vi "CompareTrackerBiasZ.vi"() -> ()   [LabVIEW 2011]
uses:
  qtrk/QTrkLVBinding/XYZf.ctl
  qtrk/lv/CPUTrkAPI.llb/TrackerDLL.vi
panel:
  out "LV LUT size":i32[](array[numeric])
  out "iz":T1(graph)
  out "iz-z":T2(graph)
  out "Error curves":dbl[][](graph)
  out "LV BestIndex":i32
  out "QTrk bestIndex":i32
  out "Profiles":sgl[][](graph)
  in  "FFT Z compare?":bool
  out "X":T2(graph)
  out "LV LUT":dbl[][](graph)
  in  "file (use dialog)":path=path "D:/jcnossen1/datasets/refbeadmagtestlutpos/experim/rotation+forceramp/exp_qi.radialzlut"
  in  "LUT":sgl[][][](array[numeric])
  out "Z":T2(graph)
  out "Z":dbl[][](graph)
  out "Image":sgl[][](graph)
  out "X":dbl[][](graph)
  out "iteration":i32
  out "Intensity Graph":sgl[][](graph)
  in  "tracker DLL path":path=path "D:/jcnossen1/cudaqi-tracker/qtrk/lv/qtrk-labview.dll"
  in  "# images":i32=1000
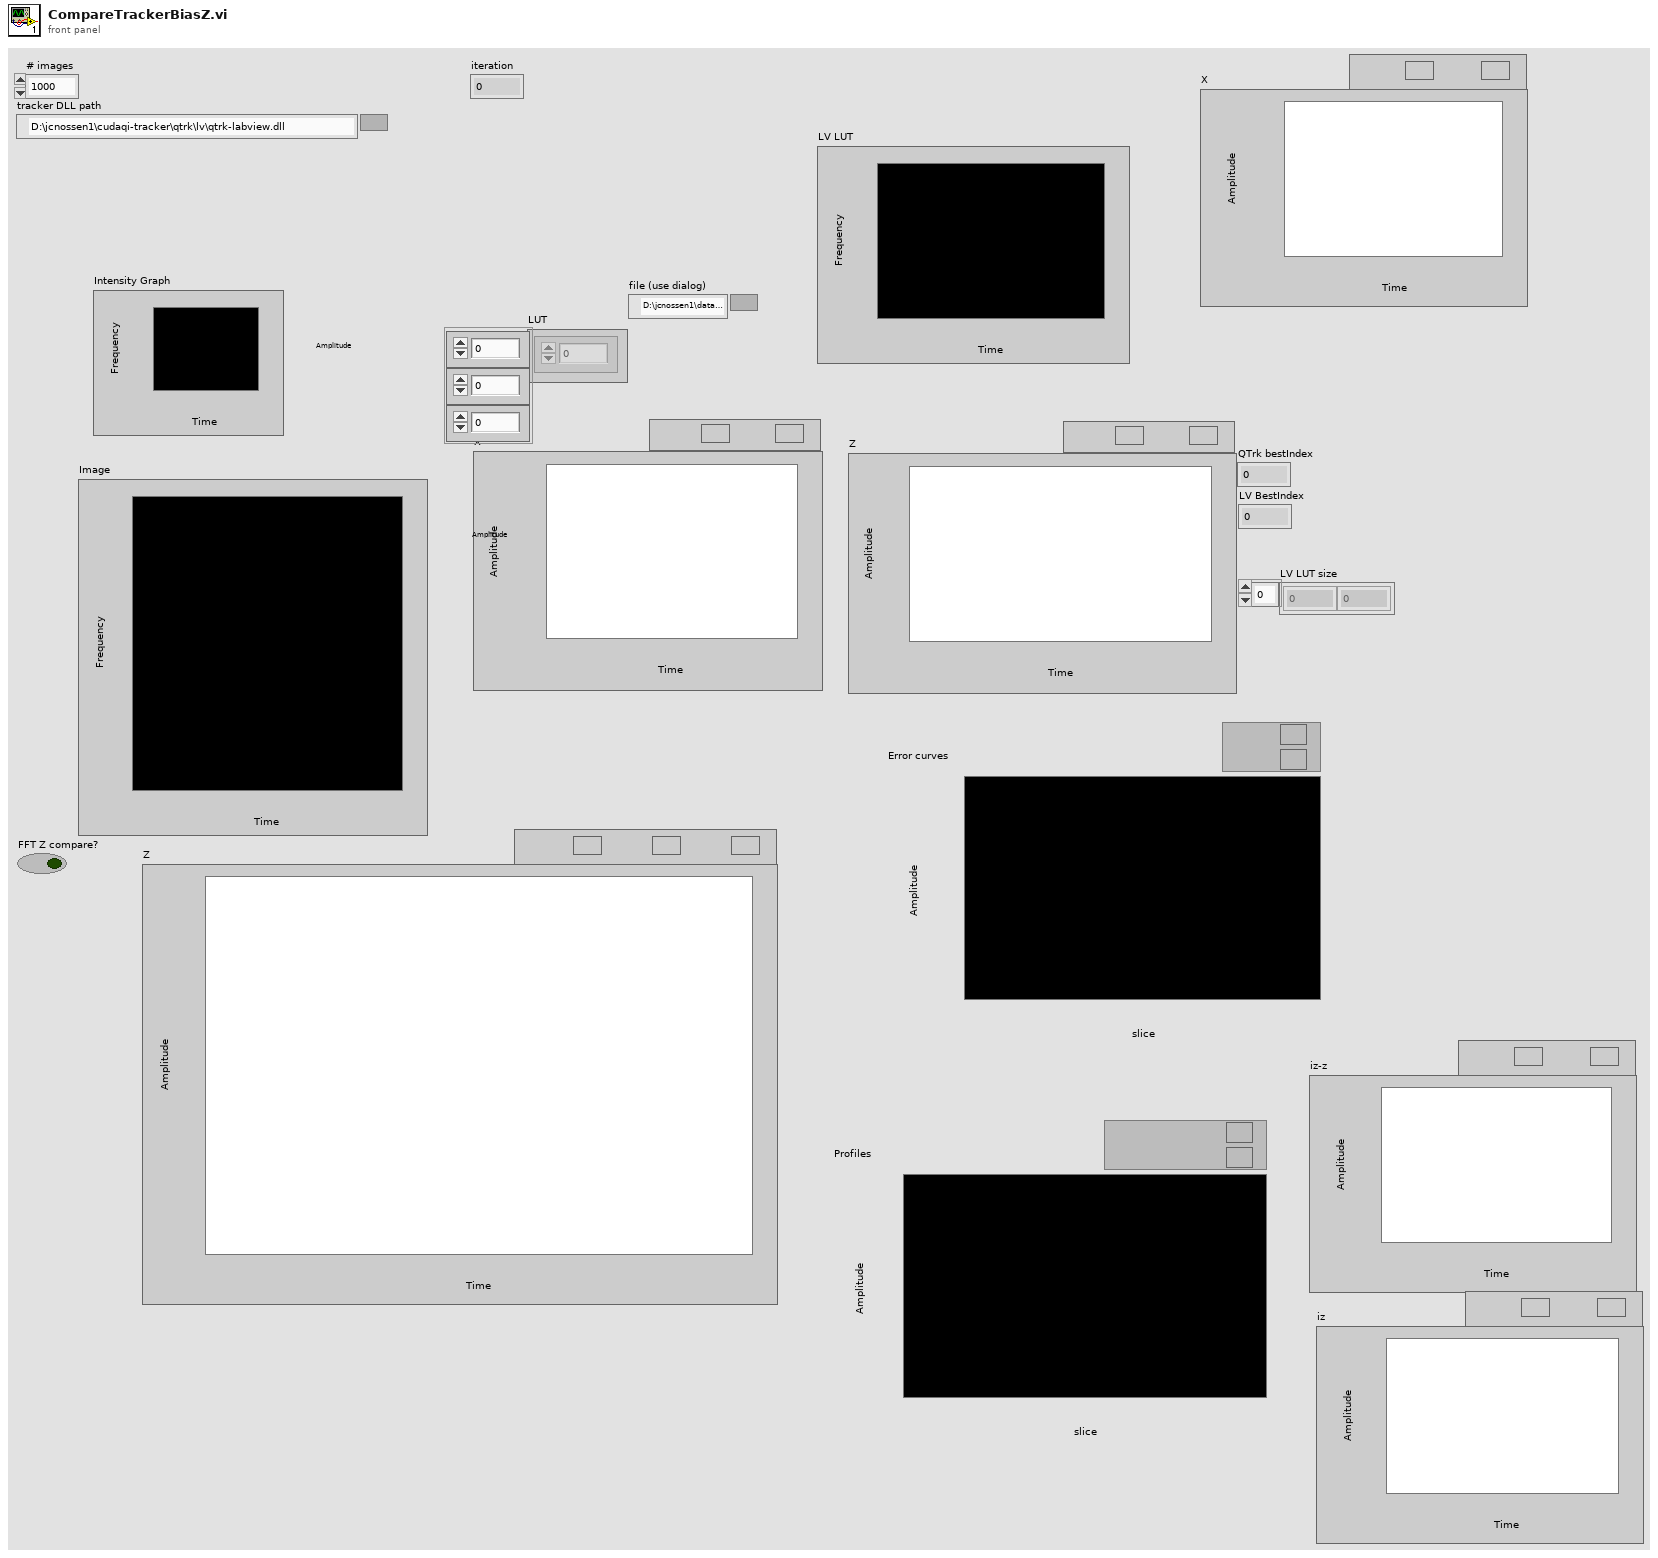
[diagram p1: front panel]
types:
  T1 = cluster{"[0]":i32, "[1]":i32, "[2]":i32, "[3]":i32, "[4]":i32, "[5]":i32, "[6]":i32, "[7]":i32, "[8]":i32}
  T2 = cluster{"[0]":dbl, "[1]":dbl, "[2]":dbl, "[3]":dbl, "[4]":dbl, "[5]":dbl, "[6]":dbl, "[7]":dbl, "[8]":dbl}
  T3 = enum16{"big-endian, network order", "native, host order", "little-endian"}
  T4 = typedef "TrackerInstance.ctl" = cluster{"Tracker Pointer":u64, "Image size":cluster{"width":u32, "height":u32}}
  T5 = cluster{"Rmax (pix)":i32, "RminZ (pix)":i32, "angular pixel\n coverage factor":dbl, "radial pixel\n coverage factor":dbl}
  T6 = typedef "XYZf.ctl" = cluster{"X":sgl, "Y":sgl, "Z":sgl}
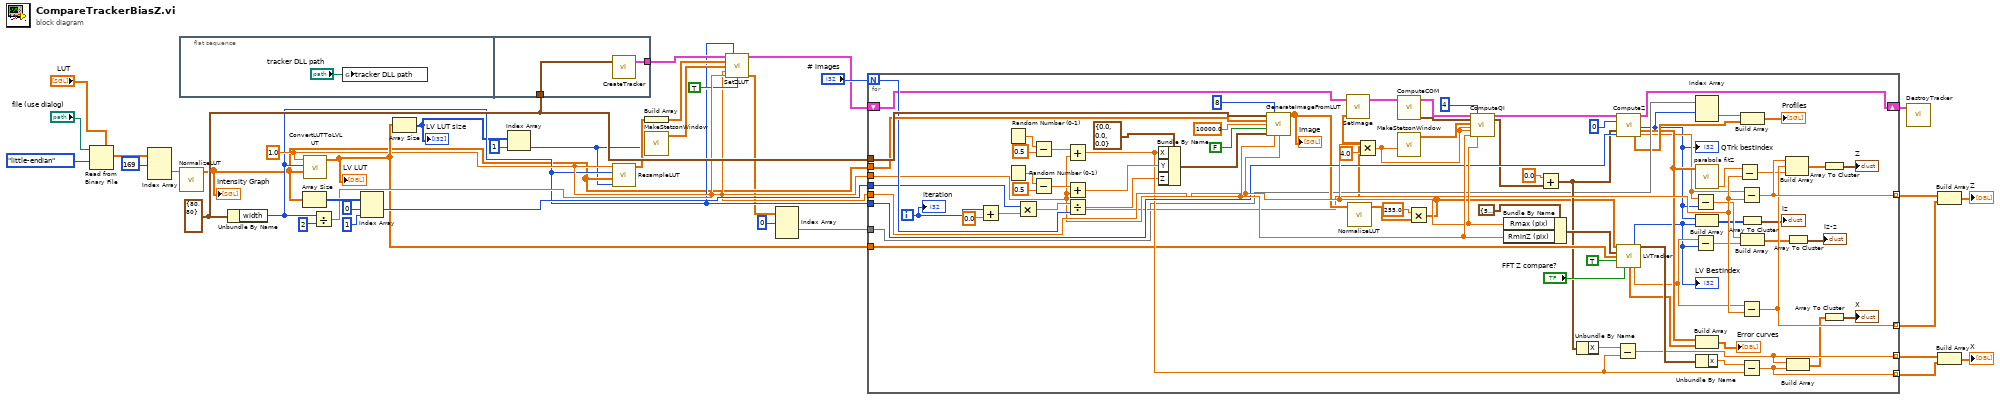
[diagram p0: block diagram]
diagram:
  w8 = sgl 1.0 ("minRadius")
  w16 = cluster{"width":u32, "height":u32} {"width"=80, "height"=80} ("Image size")
  n1 = Read from Binary File(5:"LUT", 9:T3."little-endian" ("byte order (0:big-endian, network order)"), 11:"file (use dialog)") -> (2:w19:sgl[][][])  [unwired: 3 in, 3 out]
  n2 = Index Array(array=w19, index (dim 0)=169 ("index (page)")) -> (element=w14:sgl[][])  [unwired: 2 in]
  n3 = flat-sequence {
    tunnel: [w40] -> w31
    tunnel: w16 -> [w39]
    frame #0 {
      n4 = global write "TrackerDLL.vi" "tracker DLL path"("tracker DLL path") -> ()
    }
    frame #1 {
      n5 = call "CreateTracker.vi"("Image size"=w39) -> ("tracker"=w40:T4)  [unwired: 2 in]
    }
  }
  n6 = call "NormalizeLUT.vi"("LUT"=w14) -> ("Array"=w4:sgl[][])  [unwired: 10 in]
  "Intensity Graph" <- w4
  n7 = Unbundle By Name(w16) -> ("width"=w7:u32)
  n8 = Array Size(array=w4) -> (size(s)=w35:i32[])
  n9 = call "ConvertLUTToLVLUT.vi"("LUT"=w4, "width"=w7, "minRadius"=w8) -> ("LV tracker rad prof"=w9:dbl[][])  [unwired: 8 in]
  "LV LUT" <- w9
  n10 = Divide(x=w7, y=u32 2) -> (x/y=w15:dbl)
  n11 = Index Array(array=w35, index #1=0 ("index"), index #2=1 ("index")) -> (element #1=w33:i32)  [unwired: 1 out]
  n12 = Array Size(array=w9) -> (size(s)=w6:i32[])
  "LV LUT size" <- w6
  n13 = Index Array(array=w6, index=1) -> (element=w2:i32)
  n14 = call "ResampleLUT.vi"("radialsteps"=w2, "LUT"=w4, "width"=w7, "minRadius"=w8) -> ("LUT"=w3:dbl[][])  [unwired: 7 in]
  n15 = Build Array(w3) -> (w13:dbl[][][])
  n16 = call "MakeStetsonWindow.vi"("radialsteps"=w2) -> ("Window"=w17:dbl[])  [unwired: 10 in]
  n17 = call "SetZLUT.vi"("tracker instance"=w31, "angularSteps"=w7, "zluts"=w13, "Radial weights"=w17, "minradius"=w8, "maxradius"=w15, "Normalize"=TRUE) -> ("tracker"=w30:T4, "normalized zlut"=w1:sgl[][][])  [unwired: 7 in]
  n18 = Index Array(array=w1, index (dim 0)=0 ("index (page)")) -> (element=w11:sgl[][])  [unwired: 2 in]
  n19 = for {
    N: "# images" -> [w113]
    tunnel: w16 -> [w118]
    tunnel: w4 -> [w117]
    tunnel: w15 -> [w86]
    tunnel: w33 -> [w94]
    shift-right: [w83] -> w32
    shift-left: w30 -> [w109]
    tunnel: [w70] -> w26 mode=indexing
    tunnel: [w60] -> w28 mode=indexing
    tunnel: w8 -> [w93]
    tunnel: w7 -> [w81]
    tunnel: [w79] -> w25 mode=indexing
    tunnel: [w78] -> w24 mode=indexing
    tunnel: w9 -> [w72]
    tunnel: w11 -> [w58]
    i -> [w112]
    n20 = Add(x=w112, y=0.0 ("X Range")) -> (x+y=w110:dbl)
    n21 = Random Number (0-1)() -> (number: 0 to 1=w92:dbl)
    n22 = Random Number (0-1)() -> (number: 0 to 1=w89:dbl)
    n23 = Multiply(x=w94, y=w110) -> (x*y=w114:dbl)
    n24 = Subtract(x=w92, y=0.5) -> (x-y=w90:dbl)
    n25 = Subtract(x=w89, y=0.5) -> (x-y=w87:dbl)
    n26 = Add(x=w90, y=w86) -> (x+y=w80:dbl)
    n27 = Add(x=w87, y=w86) -> (x+y=w85:dbl)
    n28 = Divide(x=w114, y=w113) -> (x/y=w63:dbl)
    n29 = Bundle By Name(cluster=T6 {"X"=0.0, "Y"=0.0, "Z"=0.0} ("XYZ"), "X"=w80, "Y"=w85, "Z"=w63) -> (w108:T6)
    n30 = call "GenerateImageFromLUT.vi"("Image Size"=w118, "samplesPerPixel"=8, "ZLUT"=w117, "Pixel max value"=sgl 10000.0, "Use spline interpolation?"=FALSE, "XYZ"=w108, "ZLUT MinRadius"=w93, "ZLUT MaxRadius"=w86) -> ("Result image"=w67:sgl[][])  [unwired: 7 in]
    "Image" <- w67
    n31 = call "NormalizeLUT.vi"("LUT"=w67) -> ("Array"=w65:sgl[][])  [unwired: 10 in]
    n32 = Multiply(x=w86, y=4.0) -> (x*y=w96:dbl)
    n33 = call "MakeStetsonWindow.vi"("radialsteps"=w96) -> ("Window"=w95:dbl[])  [unwired: 10 in]
    n34 = Multiply(x=255.0, y=w65) -> (x*y=w41:dbl[][])
    n35 = call "SetImage.vi"("tracker"=w109, "Image (float)"=w41) -> ("tracker"=w107:T4)  [unwired: 6 in, 1 out]
    n36 = call "ComputeCOM.vi"("tracker"=w107) -> ("position"=w105:cluster{"X":sgl, "Y":sgl}, "tracker"=w106:T4)  [unwired: 5 in]
    n37 = call "ComputeQI.vi"("tracker"=w106, "initial position"=w105, "radial weights (such as stetson window)"=w95, "radialSteps"=w96, "angularStepsPerQuadrant"=w96, "minRadius"=w93, "iterations"=4, "maxRadius"=w86) -> ("tracker"=w84:T4, "position"=w71:cluster{"X":sgl, "Y":sgl})  [unwired: 9 in, 1 out]
    n38 = Bundle By Name(cluster=T5 {"Rmax (pix)"=50, "RminZ (pix)"=5, "angular pixel\n coverage factor"=0.7, "radial pixel\n coverage factor"=3.0} ("settings"), "Rmax (pix)"=w86, "RminZ (pix)"=w93) -> (w101:T5)
    n39 = Add(x=0.0 ("y"), y=w71) -> (x+y=w59:cluster{"X":dbl, "Y":dbl})
    n40 = Unbundle By Name(w59) -> ("X"=w98:dbl)
    n41 = Subtract(x=w98, y=w80) -> (x-y=w70:dbl)
    n42 = call "ComputeZ.vi"("tracker instance"=w84, "zlutIndex"=0, "position"=w59, "angular_steps"=w81) -> ("tracker instance"=w83:T4, "bestIndex"=w42:i32, "errorcurve"=w54:sgl[], "dbgProfile"=w56:sgl[], "Z"=w49:sgl)  [unwired: 6 in, 1 out]
    "QTrk bestIndex" <- w42
    n43 = call "LVTracker.vi"("image in"=w41, "settings"=w101, "Z LUT"=w72, "Compute Z"=TRUE, "FFT Z compare?"="FFT Z compare?") -> ("bestLutIndex"=w43:i32, "qi position"=w100:cluster{"x":dbl, "y":dbl}, "difference"=w53:dbl[], "Z plane index"=w51:dbl)  [unwired: 3 in, 4 out]
    "LV BestIndex" <- w43
    n44 = Subtract(x=w49, y=w42) -> (x-y=w48:sgl)
    n45 = Subtract(x=w51, y=w43) -> (x-y=w50:dbl)
    n46 = Index Array(array=w58, index (row)=w42) -> (element=w57:sgl[])  [unwired: 1 in]
    n47 = call "parabola fitZ.vi"("radial profile"=w54) -> ("Y focus"=w62:dbl)  [unwired: 7 in]
    n48 = Build Array(w42, w43) -> (w44:i32[])
    n49 = Build Array(w54, w53) -> (→"Error curves":dbl[][])
    n50 = Unbundle By Name(w100) -> ("x"=w99:dbl)
    n51 = Subtract(x=w62, y=w63) -> (x-y=w61:dbl)
    n52 = Subtract(x=w49, y=w63) -> (x-y=w79:dbl)
    n53 = Subtract(x=w51, y=w63) -> (x-y=w78:dbl)
    n54 = Subtract(x=w99, y=w80) -> (x-y=w60:dbl)
    n55 = Build Array(w57, w56) -> (→"Profiles":sgl[][])
    n56 = Array To Cluster(array=w44) -> (cluster=→"iz":T1)
    n57 = Build Array(w48, w50) -> (w47:dbl[])
    n58 = Build Array(w79, w78, w61) -> (w77:dbl[])
    n59 = Array To Cluster(array=w47) -> (cluster=→"iz-z":T2)
    n60 = Build Array(w70, w60) -> (w69:dbl[])
    n61 = Array To Cluster(array=w77) -> (cluster=→"Z":T2)
    n62 = Array To Cluster(array=w69) -> (cluster=→"X":T2)
    "iteration" <- w112
  }
  n63 = call "DestroyTracker.vi"("tracker instance"=w32) -> ()  [unwired: 5 in]
  n64 = Build Array(w25, w24) -> (→"Z":dbl[][])
  n65 = Build Array(w26, w28) -> (→"X":dbl[][])
